vi "Button_Light.vi"   [LabVIEW 2012]
types:
  T1 = typedef "BotSpeak_Control.ctl" = cluster{"Address":string, "Reply EOF":string, "Hardware":string, "Retries":i8, "Timeout":i32}
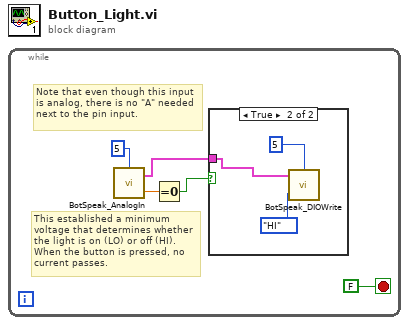
[diagram p0: block diagram]
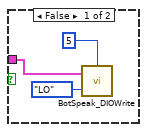
[diagram p2: hidden frame]
diagram:
  n1 = while {
    stop <- FALSE stop-if-true
    # "This established a minimum voltage that determines whether the light is on (LO) or off (HI). When the button is pressed, no current passes."
    # "Note that even though this input is analog, there is no \"A\" needed next to the pin input."
    n2 = call <userlib>:"BotSpeak_AnalogIn.vi"("A/D Channel"=u32 5 ("DIO Line")) -> ("voltage"=w2:dbl, "Bot Settings"=w5:T1)  [unwired: 2 in]
    n3 = Equal To 0?(x=w2) -> (x = 0?=w1:bool)
    n4 = case shown="True" w1 {
      tunnel: w5 -> [w6 w9]
      frame False {
        n5 = call <userlib>:"BotSpeak_DIOWrite.vi"("State"=enum32{"LO", "HI"}."LO", "Bot Settings"=w6, "DIO Line"=u32 5) -> ()  [unwired: 2 out]
      }
      frame True {
        n6 = call <userlib>:"BotSpeak_DIOWrite.vi"("State"=enum32{"LO", "HI"}."HI", "Bot Settings"=w9, "DIO Line"=u32 5) -> ()  [unwired: 2 out]
      }
    }
  }
